vi "DQMH Obtain Default Broadcast Events.vi"(7 "Path to module directory":path, 8 "error in (no error)":errorcluster, 11 "Application reference":refnum<vi>) -> (0 "error out":errorcluster, 1 "Update Module Execution Status":refnum<user-event>, 2 "Error Reported":refnum<user-event>, 3 "Status Updated":refnum<user-event>, 4 "System Message":refnum<user-event>, 5 "Module Did Stop":refnum<user-event>)   [LabVIEW 2014, in "hse-dqmh-dynamicrequesters.lvlib"]
doc: "Calls the \"Obtain Default Broadcast Events\" request VI of the module in <b>path</b>\n\n____\nHAMPEL SOFTWARE ENGINEERING v0.7.0 (2018-07-16 18:12)"
uses:
  hse-dqmh-dynamicrequesters.lvlib
  Stop Argument--cluster.ctl
  Status Updated Argument--cluster.ctl
  Error Reported Argument--cluster.ctl
  Get Module Execution Status Argument--cluster.ctl
  Controls/System Message Argument--cluster.ctl
  Controls/System Message Source.ctl
  hse-dqmh.lvlib
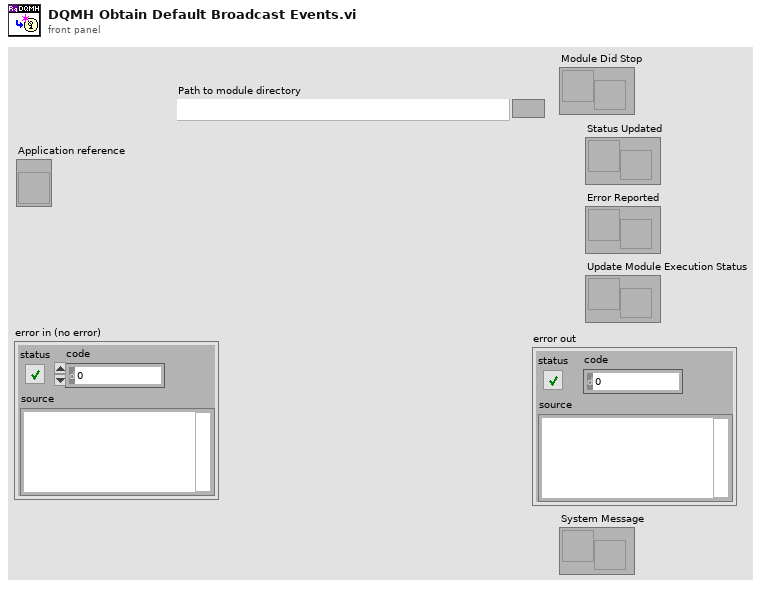
[diagram p1: front panel]
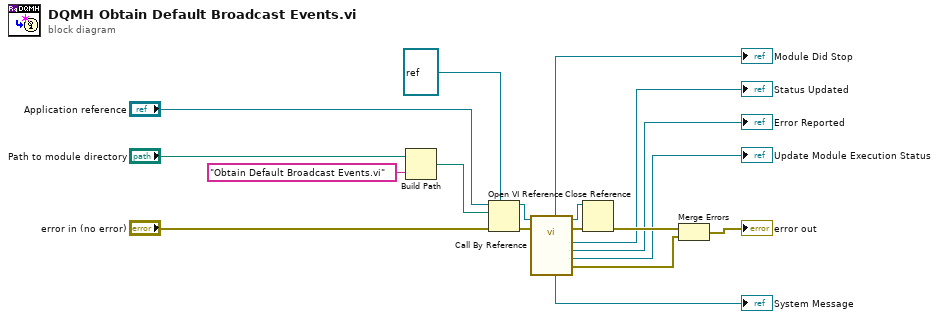
[diagram p0: block diagram]
diagram:
  n1 = Build Path(base path="Path to module directory", name or relative path="Obtain Default Broadcast Events.vi") -> (appended path=w7:path)
  n2 = Open VI Reference(type specifier VI Refnum (for type only)=refnum<vi> refnum, application reference (local)="Application reference", vi path=w7, error in (no error)="error in (no error)") -> (vi reference=w13:refnum<vi>, error out=w14:errorcluster)  [unwired: 2 in]
  n3 = call-by-ref "?"(reference=w13, error in=w14) -> (reference out=w11:refnum<vi>, error out=w12:errorcluster, 0:"error out"=w6:errorcluster, "Update Module Execution Status"=→"Update Module Execution Status":refnum<user-event>, "Error Reported"=→"Error Reported":refnum<user-event>, "Status Updated"=→"Status Updated":refnum<user-event>, "System Message"=→"System Message":refnum<user-event>, "Module Did Stop"=→"Module Did Stop":refnum<user-event>)  [unwired: 6 in]
  n4 = Close Reference(reference=w11, error in (no error)=w12) -> (error out=w10:errorcluster)
  n5 = Merge Errors(w10, w6) -> (→"error out":errorcluster)
